vi "Setmsg_2.vi"(8 "error in (no error)":errorcluster, 10 "Set_Val":T1, 11 "OneOfTemplate in":refnum<class "w4lvgrpc_ToClient_payload.lvclass">) -> (0 "error out":errorcluster, 3 "OneOfTemplate out":refnum<class "w4lvgrpc_ToClient_payload.lvclass">)   [LabVIEW 2019, in "Generated_client.lvlib" / "w4lvgrpc_ToClient_payload.lvclass"]
uses:
  w4lvgrpc_ToClient_payload.lvclass
  w4lvgrpc_Msg_ToClient_2.ctl
  Generated_client.lvlib
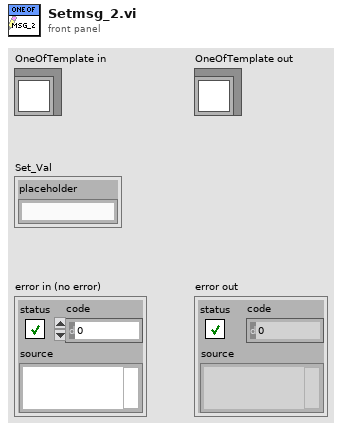
[diagram p1: front panel]
types:
  T1 = typedef "Generated_client.lvlib/w4lvgrpc_Msg_ToClient_2.ctl" = cluster{"placeholder":string}
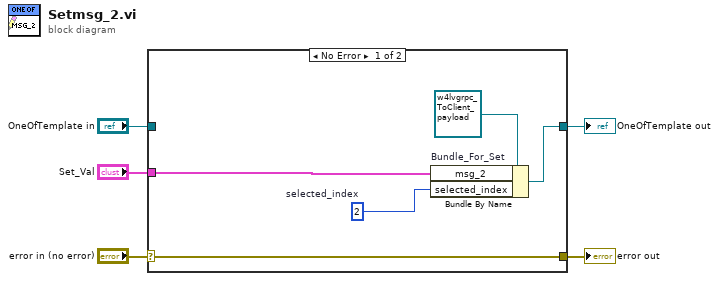
[diagram p0: block diagram]
diagram:
  n1 = case shown="No Error" "error in (no error)" {
    selector: "error in (no error)" -> [w10 w11]
    tunnel: [w10 w11] -> w4
    tunnel: [w9 w12] -> w2
    tunnel: "OneOfTemplate in" -> [_ w12]
    tunnel: "Set_Val" -> [w8 _]
    frame No Error {
      w7 = 2  # selected_index
      n2 = Bundle By Name "Bundle_For_Set"(cluster=refnum<class "w4lvgrpc_ToClient_payload.lvclass"> refnum ("OneOfTemplate in"), "msg_2"=w8, "selected_index"=w7) -> (w9:refnum<class "w4lvgrpc_ToClient_payload.lvclass">)
    }
    frame Error {
    }
  }
  "error out" <- w4
  "OneOfTemplate out" <- w2
